vi "Simulador Circuito RLC.Final- Gullit e Gabriela.vi"() -> ()   [LabVIEW 2020]
uses:
  <vilib>/Utility/file.llb/Read Delimited Spreadsheet (DBL).vi
  <vilib>/measure/NI_MABase.lvlib
panel:
  in  "i'(0)":dbl=1.0
  in  "i(0)":dbl
  in  "Vc'(0)":dbl=1.0
  in  "Vc(0)":dbl
  in  "C":dbl
  in  "L":dbl
  in  "R":dbl
  in  "Gerar ondas\nde saída":bool
  out "Tensão no Capacitor":cluster{dbl[], "Y":dbl[]}[](graph)
  out "Corrente":cluster{dbl[], "Y":dbl[]}[](graph)
  in  "Arquivo texto da onda":path
  out "Onda de entrada":cluster{dbl[], "Y":dbl[]}(graph)
  in  "Duty Cicle":dbl
  in  "Informação da amostragem":T1={"Taxa de amostragem"=1000.0, "N° de amostras"=10000.0} {"N° de amostras" format="%#.6g"; "Taxa de amostragem" format="%#.6g"}
  in  "Gerar onda \nde Entrada":bool
  in  "Tipo de Onda":u16(ring) items=["Senoidal", "Quadrada", "Onda qualquer", ""]
  in  "Amplitude":dbl
  in  "Frequência":dbl
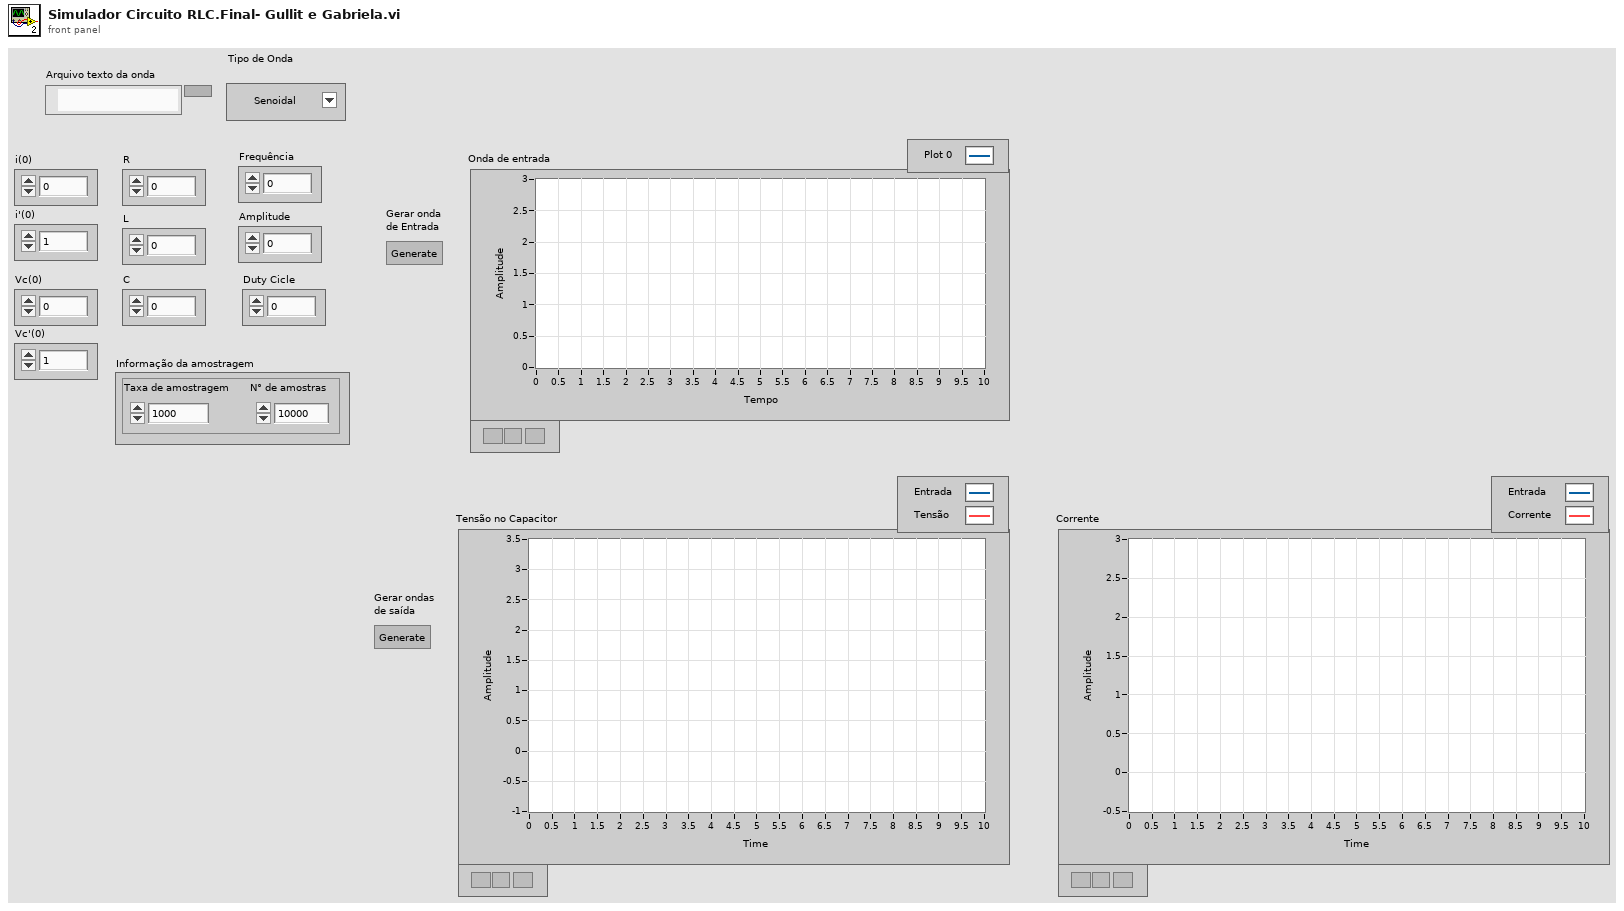
[diagram p1: front panel]
types:
  T1 = cluster{"Taxa de amostragem":dbl, "N° de amostras":dbl}
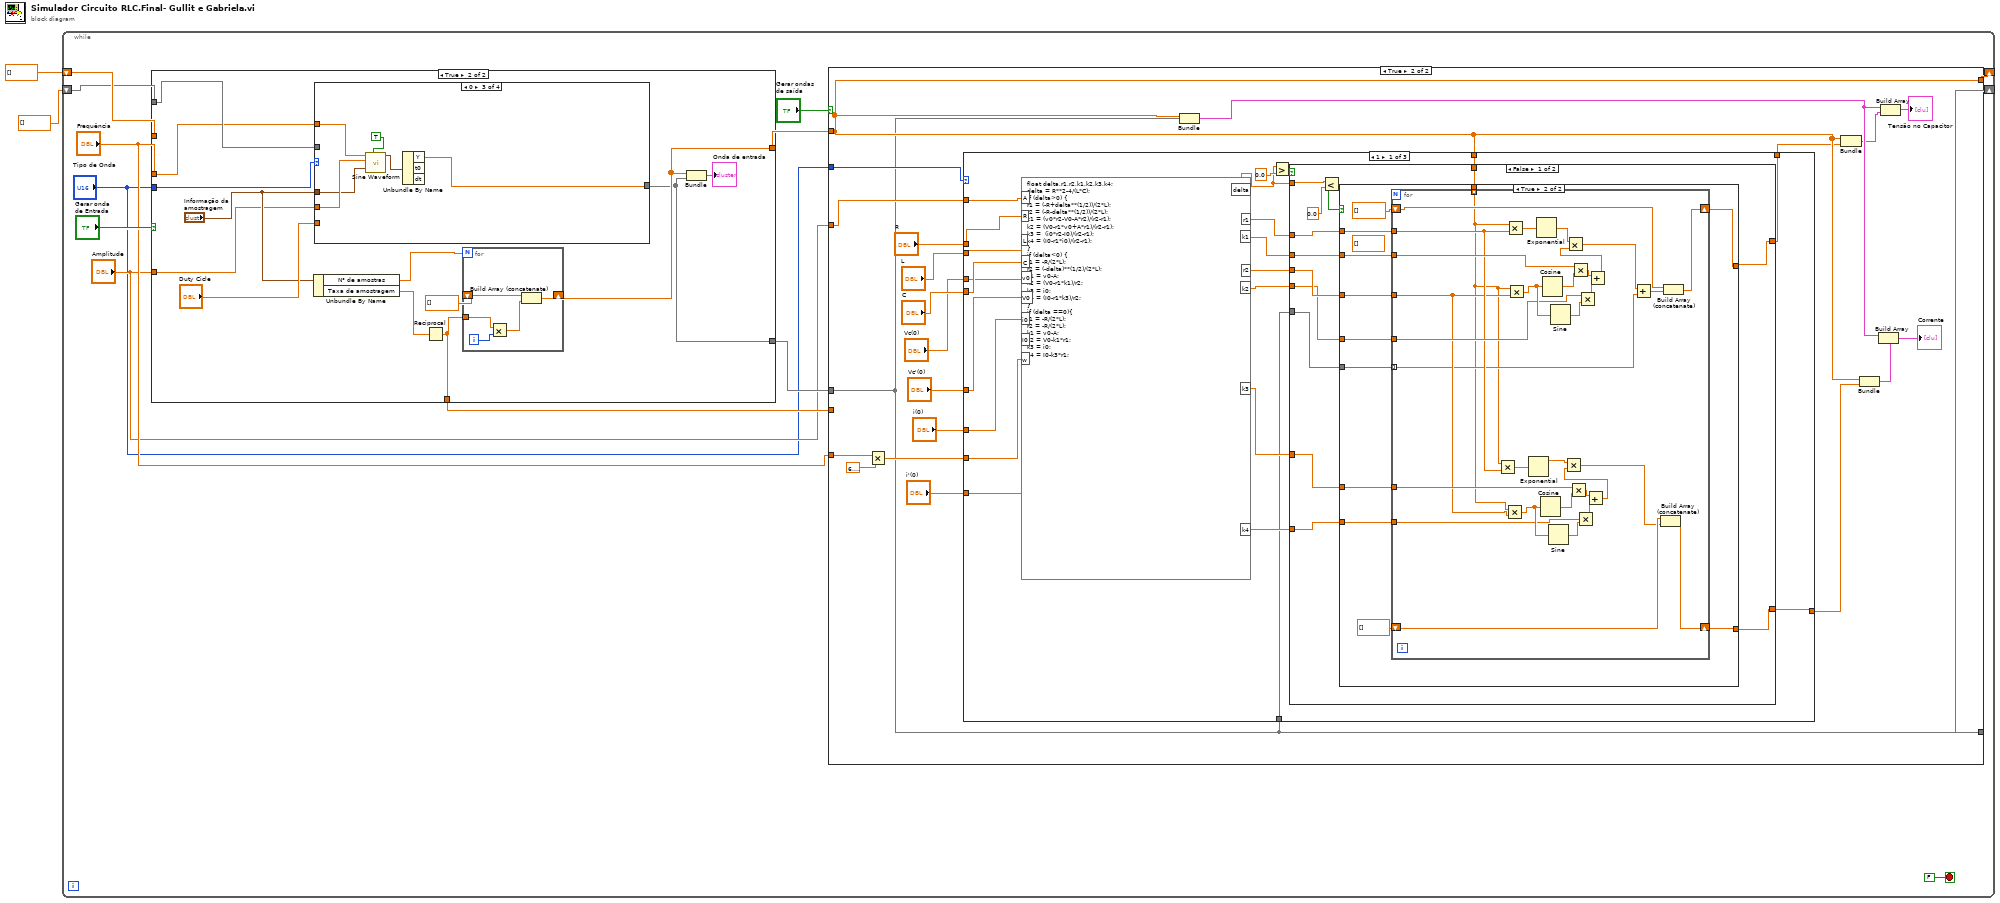
[diagram p0: block diagram]
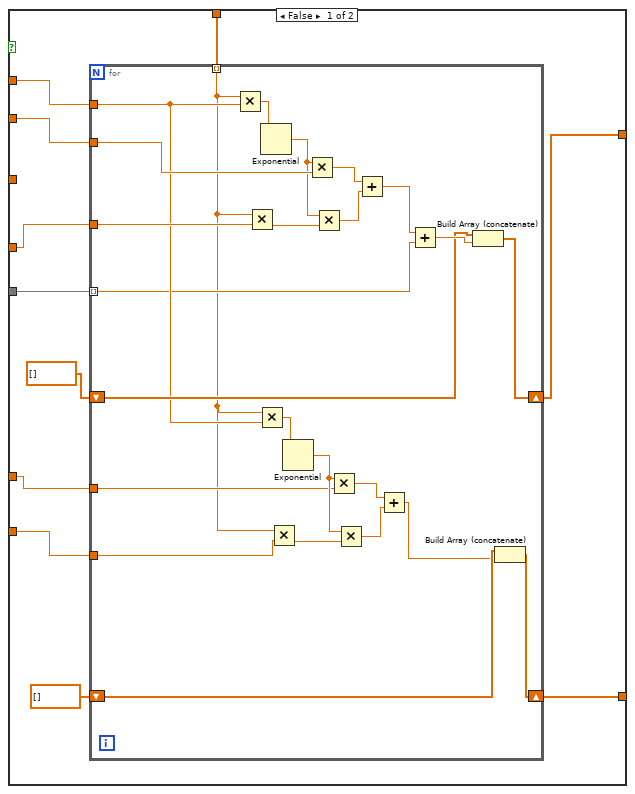
[diagram p3: hidden frame]
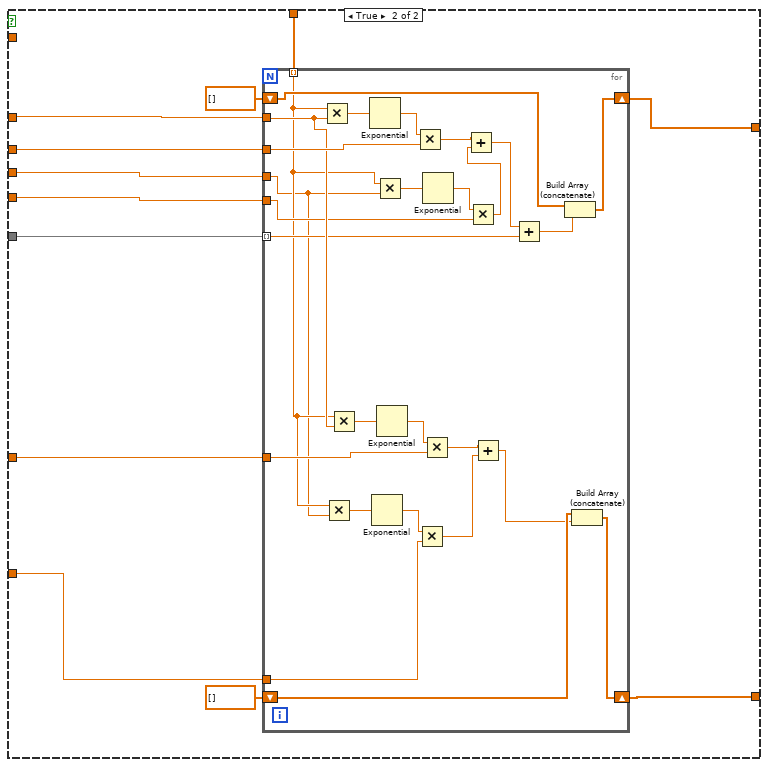
[diagram p4: hidden frame]
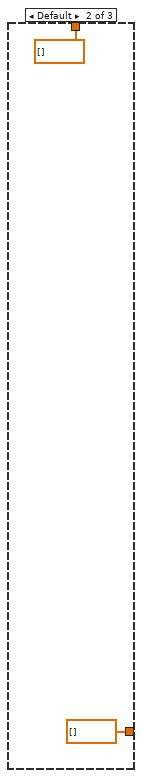
[diagram p5: hidden frame]
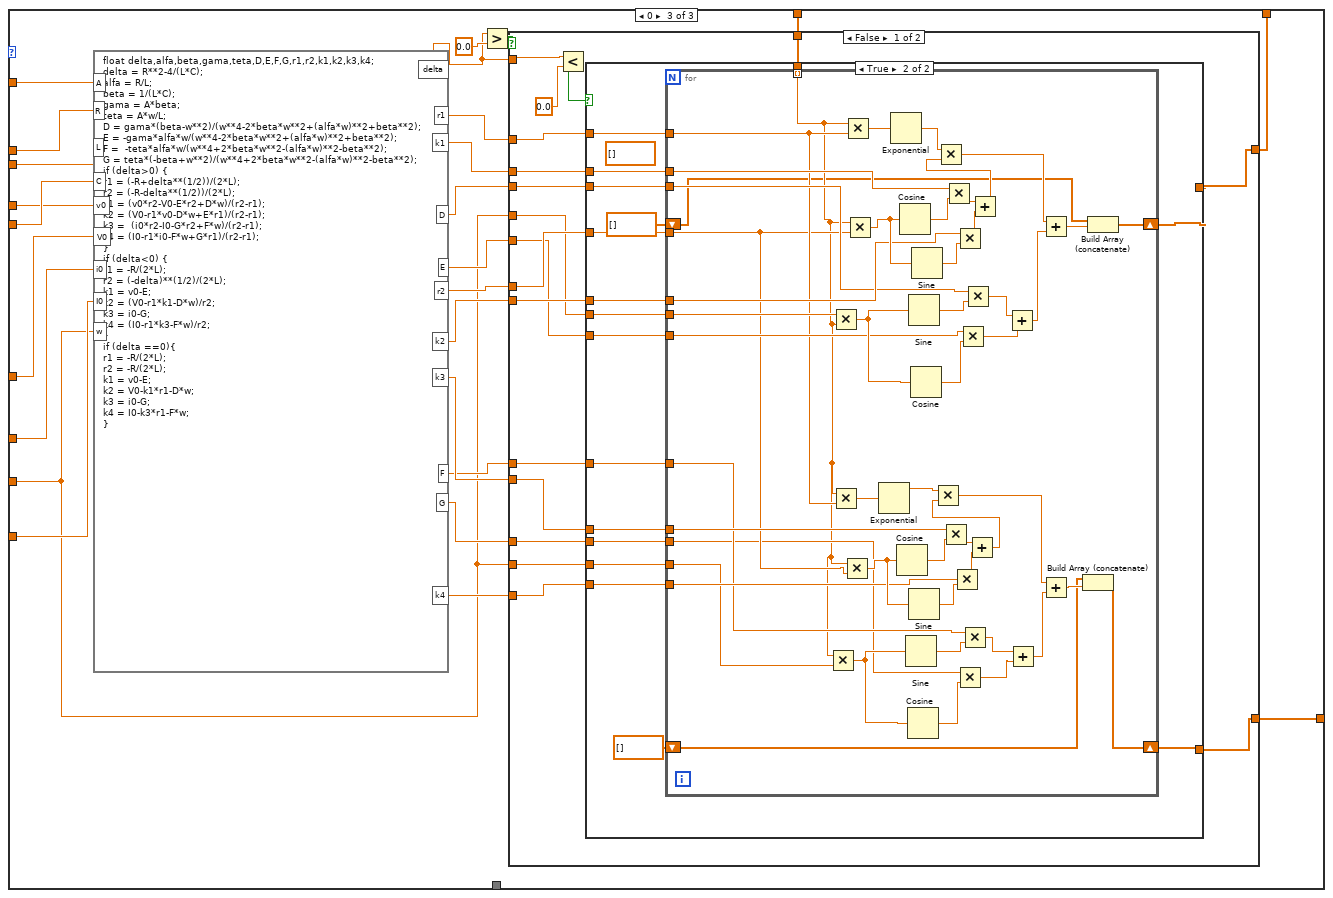
[diagram p6: hidden frame]
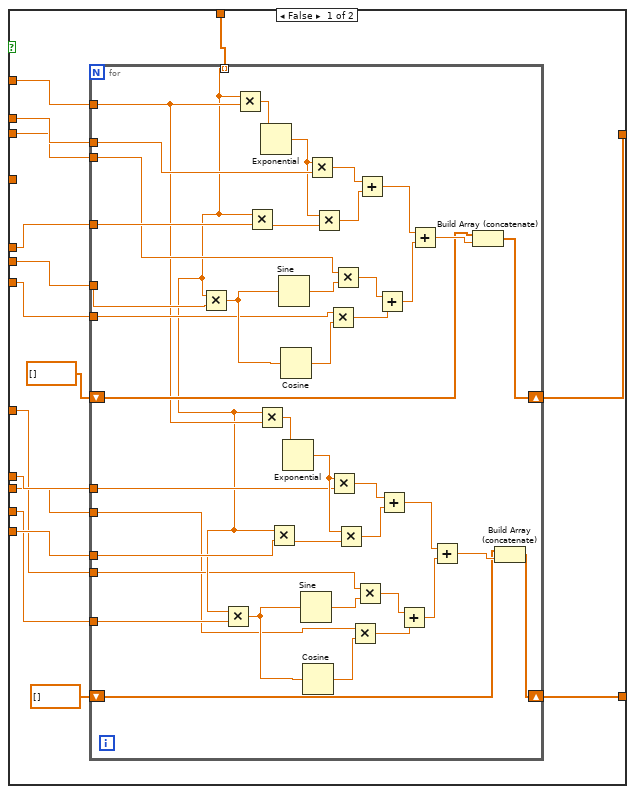
[diagram p7: hidden frame]
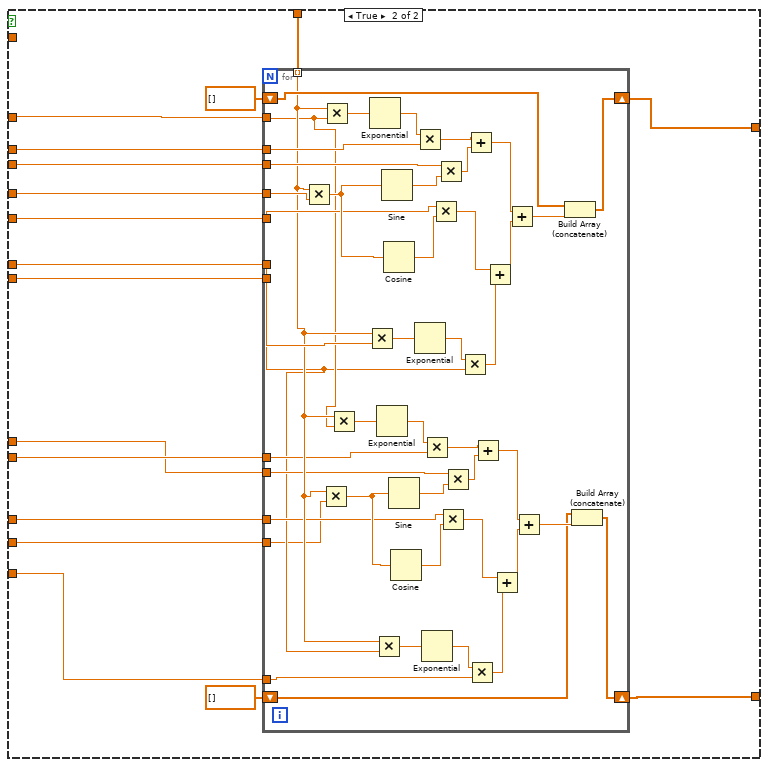
[diagram p8: hidden frame]
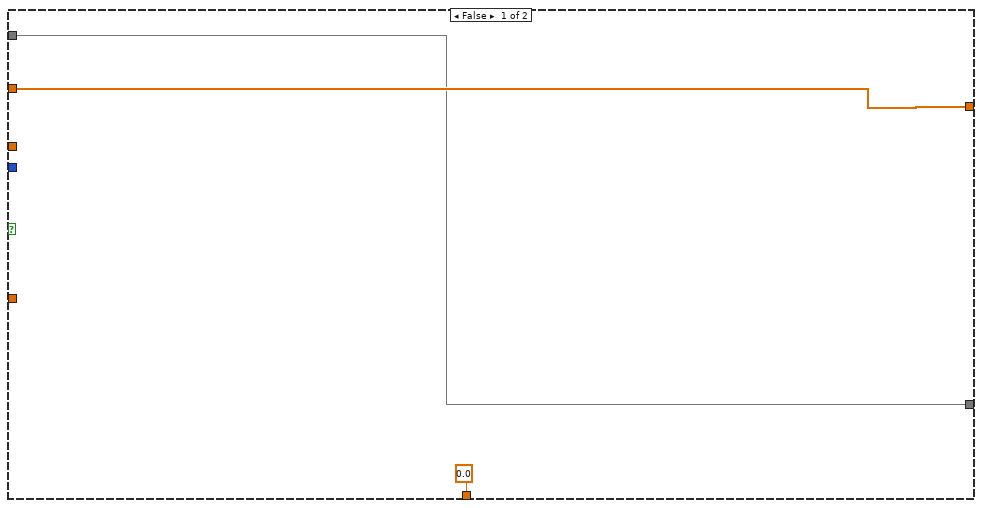
[diagram p9: hidden frame]
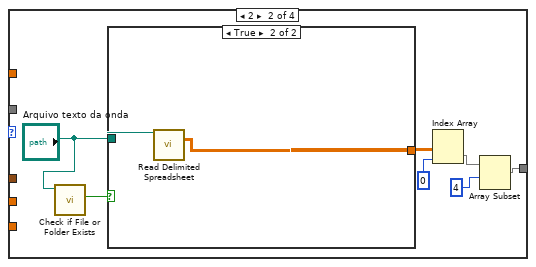
[diagram p11: hidden frame]
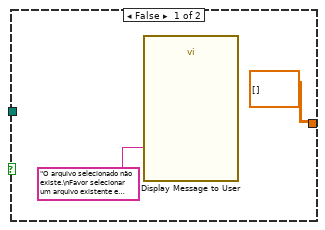
[diagram p12: hidden frame]
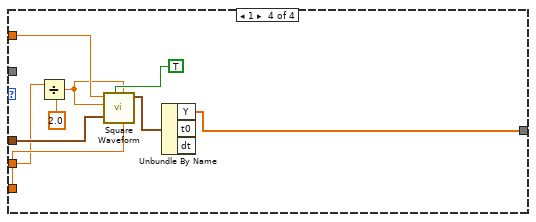
[diagram p13: hidden frame]
diagram:
  n1 = while {
    shift-right: [w11] -> _
    shift-left: dbl[] [] -> [w9]
    shift-right: [w10] -> _
    shift-left: dbl[] [] ("Y") -> [w8]
    stop <- FALSE stop-if-true
    n2 = case shown="True" "Gerar onda \nde Entrada" {
      tunnel: [w424 w432] -> w13
      tunnel: [w423 w431] -> w12
      tunnel: w9 -> [w424 _]
      tunnel: w8 -> [w423 w430]
      tunnel: [0.0 w428] -> w7
      tunnel: "Frequência" -> [_ w427]
      tunnel: "Amplitude" -> [_ w426]
      tunnel: "Tipo de Onda" -> [_ w425]
      frame False {
      }
      frame True {
        n3 = Unbundle By Name("Informação da amostragem") -> ("N° de amostras"=w434:dbl, "Taxa de amostragem"=w435:dbl)
        n4 = case shown="0" w425 {
          tunnel: w426 -> [_ _ w459 w462]
          tunnel: w427 -> [_ _ w460 w469]
          tunnel: w430 -> [w443 _ _ _]
          tunnel: "Informação da amostragem" -> [_ _ w458 w468]
          tunnel: "Duty Cicle" -> [_ _ _ w467]
          tunnel: [w443 w446 w455 w464] -> w431
          frame Default {
          }
          frame 2 {
            n5 = call <vilib>:"Check if File or Folder Exists.vi"("path"="Arquivo texto da onda") -> ("file or folder exists?"=w444:bool)  [unwired: 8 in, 2 out]
            n6 = case shown="True" w444 {
              tunnel: "Arquivo texto da onda" -> [_ w454]
              tunnel: [dbl[][] [] ("all rows") w453] -> w448
              frame False {
                n7 = call "Display Message to User"("Message"="O arquivo selecionado não existe.\nFavor selecionar um arquivo existente e recomeçe a VI.") -> ()  [unwired: 9 in, 2 out]
              }
              frame True {
                n8 = call-poly <vilib>:"Read Delimited Spreadsheet.vi"("file path (dialog if empty)"=w454) -> ("all rows"=w453:dbl[][])  [unwired: 9 in, 5 out]
              }
            }
            n9 = Index Array(array=w448, index (col)=0 ("disabled index (col)")) -> (element=w449:dbl[])  [unwired: 1 in]
            n10 = Array Subset(array=w449, index=4) -> (w446:dbl[])  [unwired: 1 in]
          }
          frame 0 {
            n11 = call <vilib>:"Sine Waveform.vi"("sampling info"=w458, "reset signal"=TRUE, "amplitude"=w459, "frequency"=w460) -> ("signal out"=w456:waveform(dbl))  [unwired: 6 in, 1 out]
            n12 = Unbundle By Name(w456) -> ("Y"=w455:dbl[])  [unwired: 2 out]
          }
          frame 1 {
            n13 = Divide(x=w462, y=2.0) -> (x/y=w461:dbl)
            n14 = call <vilib>:"Square Waveform.vi"("duty cycle (%)"=w467, "offset"=w461, "sampling info"=w468, "reset signal"=TRUE, "amplitude"=w461, "frequency"=w469) -> ("signal out"=w465:waveform(dbl))  [unwired: 4 in, 1 out]
            n15 = Unbundle By Name(w465) -> ("Y"=w464:dbl[])  [unwired: 2 out]
          }
        }
        n16 = Reciprocal(x=w435) -> (1/x=w428:dbl)
        n17 = for {
          N: w434 -> [_]
          tunnel: w428 -> [w441]
          shift-right: [w439] -> w432
          shift-left: dbl[] [] -> [w438]
          i -> [w442]
          n18 = Multiply(x=w441, y=w442) -> (x*y=w440:dbl)
          n19 = Build Array (concatenate)(w438, w440) -> (w439:dbl[])
        }
        n20 = Bundle(w432, "Y"=w431) -> (→"Onda de entrada":cluster{dbl[], "Y":dbl[]})  [unwired: 1 in]
      }
    }
    n21 = case shown="True" "Gerar ondas\nde saída" {
      tunnel: w13 -> [w17 w30]
      tunnel: w12 -> [w16 w18]
      tunnel: [w17 w30] -> w11
      tunnel: [w16 w18] -> w10
      tunnel: w7 -> [_ _]
      tunnel: "Amplitude" -> [_ w20]
      tunnel: "Frequência" -> [_ w22]
      tunnel: "Tipo de Onda" -> [_ w19]
      frame False {
      }
      frame True {
        n22 = Multiply(x=w22, y=6.283185307179586) -> (x*y=w21:dbl)
        n23 = case shown="1" w19 {
          tunnel: "C" -> [w48 _ w217]
          tunnel: "L" -> [w49 _ w216]
          tunnel: "R" -> [w50 _ w215]
          tunnel: "Vc(0)" -> [w47 _ w212]
          tunnel: "Vc'(0)" -> [w46 _ w211]
          tunnel: w30 -> [w42 _ w210]
          tunnel: "i(0)" -> [w45 _ w203]
          tunnel: "i'(0)" -> [w43 _ w202]
          tunnel: [w40 dbl[] [] w196] -> w27
          tunnel: [w41 dbl[] [] w195] -> w26
          tunnel: w21 -> [w44 _ w194]
          tunnel: w20 -> [w51 _ w193]
          tunnel: w18 -> [w39 _ _]
          frame 1 {
            n24 = formula code="float delta,r1,r2,k1,k2,k3,k4;\ndelta = R**2-4/(L*C);\nif (delta>0) {\nr1 = (-R+delta**(1/2))/(2*L);\nr2 = (-R-delta**(1/2))/(2*L);\nk1 = (v0*r2-V0-A*r2)/(r2-r1);\nk2 = (V0-r1*v0+A*r1)/(r2-r1);\nk3 =  (i0*r2-I0)/(r2-r1);\nk4 = (I0-r1*i0)/(r2-r1);\n}\nif (delta<0) {\nr1 = -R/(2*L);\nr2 = (-delta)**(1/2)/(2*L);\nk1 = v0-A;\nk2 = (V0-r1*k1)/r2;\nk3 = i0;\nk4 = (I0-r1*k3)/r2;\n}\nif (delta ==0){\nr1 = -R/(2*L);\nr2 = -R/(2*L);\nk1 = v0-A;\nk2 = V0-k1*r1;\nk3 = i0;\nk4 = I0-k3*r1;\n}"("C"=w48, "L"=w49, "R"=w50, "A"=w51, "w"=w44, "v0"=w47, "V0"=w46, "i0"=w45, "I0"=w43) -> ("delta"=w52:dbl, "r1"=w58:dbl, "r2"=w56:dbl, "k1"=w57:dbl, "k2"=w55:dbl, "k3"=w54:dbl, "k4"=w53:dbl)
            n25 = Greater?(x=w52, y=0.0) -> (0:w59:bool)
            n26 = case shown="False" w59 {
              tunnel: w58 -> [w70 w163]
              tunnel: w57 -> [w69 w162]
              tunnel: w56 -> [w68 w161]
              tunnel: w55 -> [w67 w160]
              tunnel: w54 -> [w66 w158]
              tunnel: w53 -> [w65 w157]
              tunnel: w52 -> [w72 _]
              tunnel: [w63 w155] -> w40
              tunnel: [w64 w154] -> w41
              tunnel: w42 -> [w62 w153]
              tunnel: w39 -> [w61 w152]
              frame False {
                n27 = Less?(x=w72, y=0.0) -> (x < y?=w73:bool)
                n28 = case shown="True" w73 {
                  tunnel: w70 -> [w83 w120]
                  tunnel: w69 -> [w84 w119]
                  tunnel: w68 -> [_ w118]
                  tunnel: w67 -> [w82 w117]
                  tunnel: w66 -> [w80 w116]
                  tunnel: w65 -> [w79 w115]
                  tunnel: [w74 w109] -> w63
                  tunnel: [w77 w113] -> w64
                  tunnel: w62 -> [w76 w111]
                  tunnel: w61 -> [w75 w110]
                  frame False {
                    n29 = for {
                      tunnel: w84 -> [w108]
                      tunnel: w83 -> [w92]
                      tunnel: w82 -> [w106]
                      shift-right: [w99] -> w74
                      shift-left: dbl[] [] -> [w98]
                      tunnel: w80 -> [w91]
                      tunnel: w79 -> [w90]
                      shift-right: [w89] -> w77
                      shift-left: dbl[] [] -> [w88]
                      tunnel: w76 -> [w86] mode=indexing
                      tunnel: w75 -> [w87] mode=indexing
                      n30 = Multiply(x=w86, y=w92) -> (x*y=w107:dbl)
                      n31 = Multiply(x=w86, y=w106) -> (x*y=w105:dbl)
                      n32 = Multiply(x=w86, y=w92) -> (x*y=w97:dbl)
                      n33 = Exponential(1:w107) -> (0:w104:dbl)
                      n34 = Multiply(x=w86, y=w90) -> (x*y=w96:dbl)
                      n35 = Exponential(1:w97) -> (0:w95:dbl)
                      n36 = Multiply(x=w104, y=w108) -> (x*y=w103:dbl)
                      n37 = Multiply(x=w104, y=w105) -> (x*y=w102:dbl)
                      n38 = Multiply(x=w95, y=w91) -> (x*y=w94:dbl)
                      n39 = Multiply(x=w95, y=w96) -> (x*y=w93:dbl)
                      n40 = Add(x=w103, y=w102) -> (x+y=w101:dbl)
                      n41 = Add(x=w94, y=w93) -> (x+y=w85:dbl)
                      n42 = Add(x=w101, y=w87) -> (x+y=w100:dbl)
                      n43 = Build Array (concatenate)(w98, w100) -> (w99:dbl[])
                      n44 = Build Array (concatenate)(w88, w85) -> (w89:dbl[])
                    }
                  }
                  frame True {
                    (unwired) dbl[] []
                    n45 = for {
                      tunnel: w120 -> [w139]
                      tunnel: w119 -> [w147]
                      tunnel: w118 -> [w129]
                      tunnel: w117 -> [w143]
                      tunnel: w116 -> [w132]
                      tunnel: w115 -> [w131]
                      shift-right: [w127] -> w113
                      shift-left: dbl[] [] -> [w126]
                      shift-right: [w125] -> w109
                      shift-left: dbl[] [] -> [w124]
                      tunnel: w111 -> [w122] mode=indexing
                      tunnel: w110 -> [w123] mode=indexing
                      n46 = Multiply(x=w122, y=w139) -> (x*y=w148:dbl)
                      n47 = Multiply(x=w122, y=w129) -> (x*y=w137:dbl)
                      n48 = Multiply(x=w122, y=w139) -> (x*y=w151:dbl)
                      n49 = Multiply(x=w122, y=w129) -> (x*y=w145:dbl)
                      n50 = Exponential(1:w148) -> (0:w133:dbl)
                      n51 = Exponential(1:w151) -> (0:w150:dbl)
                      n52 = Cosine(x=w137) -> (cos(x)=w138:dbl)
                      n53 = Cosine(x=w145) -> (cos(x)=w146:dbl)
                      n54 = Sine(x=w137) -> (sin(x)=w136:dbl)
                      n55 = Sine(x=w145) -> (sin(x)=w144:dbl)
                      n56 = Multiply(x=w132, y=w138) -> (x*y=w135:dbl)
                      n57 = Multiply(x=w147, y=w146) -> (x*y=w142:dbl)
                      n58 = Multiply(x=w131, y=w136) -> (x*y=w134:dbl)
                      n59 = Multiply(x=w143, y=w144) -> (x*y=w141:dbl)
                      n60 = Add(x=w135, y=w134) -> (x+y=w130:dbl)
                      n61 = Multiply(x=w133, y=w130) -> (x*y=w121:dbl)
                      n62 = Add(x=w142, y=w141) -> (x+y=w140:dbl)
                      n63 = Multiply(x=w150, y=w140) -> (x*y=w128:dbl)
                      n64 = Add(x=w128, y=w123) -> (x+y=w149:dbl)
                      n65 = Build Array (concatenate)(w126, w121) -> (w127:dbl[])
                      n66 = Build Array (concatenate)(w124, w149) -> (w125:dbl[])
                    }
                  }
                }
              }
              frame True {
                n67 = for {
                  tunnel: w163 -> [w175]
                  tunnel: w162 -> [w190]
                  tunnel: w161 -> [w167]
                  tunnel: w160 -> [w171]
                  shift-right: [w182] -> w155
                  shift-left: dbl[] [] -> [w181]
                  tunnel: w158 -> [w174]
                  tunnel: w157 -> [w166]
                  shift-right: [w173] -> w154
                  shift-left: dbl[] [] -> [w172]
                  tunnel: w153 -> [w168] mode=indexing
                  tunnel: w152 -> [w169] mode=indexing
                  n68 = Multiply(x=w168, y=w175) -> (x*y=w189:dbl)
                  n69 = Multiply(x=w168, y=w167) -> (x*y=w178:dbl)
                  n70 = Multiply(x=w168, y=w175) -> (x*y=w180:dbl)
                  n71 = Exponential(1:w189) -> (0:w188:dbl)
                  n72 = Exponential(1:w178) -> (0:w177:dbl)
                  n73 = Multiply(x=w168, y=w167) -> (x*y=w187:dbl)
                  n74 = Exponential(1:w180) -> (0:w179:dbl)
                  n75 = Multiply(x=w188, y=w190) -> (x*y=w185:dbl)
                  n76 = Multiply(x=w177, y=w166) -> (x*y=w165:dbl)
                  n77 = Multiply(x=w179, y=w174) -> (x*y=w176:dbl)
                  n78 = Exponential(1:w187) -> (0:w186:dbl)
                  n79 = Multiply(x=w186, y=w171) -> (x*y=w170:dbl)
                  n80 = Add(x=w185, y=w170) -> (x+y=w184:dbl)
                  n81 = Add(x=w176, y=w165) -> (x+y=w164:dbl)
                  n82 = Add(x=w184, y=w169) -> (x+y=w183:dbl)
                  n83 = Build Array (concatenate)(w181, w183) -> (w182:dbl[])
                  n84 = Build Array (concatenate)(w172, w164) -> (w173:dbl[])
                }
              }
            }
          }
          frame Default {
          }
          frame 0 {
            n85 = formula code="float delta,alfa,beta,gama,teta,D,E,F,G,r1,r2,k1,k2,k3,k4;\ndelta = R**2-4/(L*C);\nalfa = R/L;\nbeta = 1/(L*C);\ngama = A*beta;\nteta = A*w/L;\nD = gama*(beta-w**2)/(w**4-2*beta*w**2+(alfa*w)**2+beta**2);\nE = -gama*alfa*w/(w**4-2*beta*w**2+(alfa*w)**2+beta**2);\nF =  -teta*alfa*w/(w**4+2*beta*w**2-(alfa*w)**2-beta**2);\nG = teta*(-beta+w**2)/(w**4+2*beta*w**2-(alfa*w)**2-beta**2);\nif (delta>0) {\nr1 = (-R+delta**(1/2))/(2*L);\nr2 = (-R-delta**(1/2))/(2*L);\nk1 = (v0*r2-V0-E*r2+D*w)/(r2-r1);\nk2 = (V0-r1*v0-D*w+E*r1)/(r2-r1);\nk3 =  (i0*r2-I0-G*r2+F*w)/(r2-r1);\nk4 = (I0-r1*i0-F*w+G*r1)/(r2-r1);\n}\nif (delta<0) {\nr1 = -R/(2*L);\nr2 = (-delta)**(1/2)/(2*L);\nk1 = v0-E;\nk2 = (V0-r1*k1-D*w)/r2;\nk3 = i0-G;\nk4 = (I0-r1*k3-F*w)/r2;\n}\nif (delta ==0){\nr1 = -R/(2*L);\nr2 = -R/(2*L);\nk1 = v0-E;\nk2 = V0-k1*r1-D*w;\nk3 = i0-G;\nk4 = I0-k3*r1-F*w;\n}"("C"=w217, "L"=w216, "R"=w215, "A"=w193, "w"=w194, "v0"=w212, "V0"=w211, "i0"=w203, "I0"=w202) -> ("D"=w204:dbl, "E"=w205:dbl, "delta"=w197:dbl, "r1"=w209:dbl, "r2"=w207:dbl, "k1"=w208:dbl, "k2"=w206:dbl, "k3"=w201:dbl, "k4"=w198:dbl, "F"=w200:dbl, "G"=w199:dbl)
            n86 = Greater?(x=w197, y=0.0) -> (0:w213:bool)
            n87 = case shown="False" w213 {
              tunnel: w210 -> [w232 w376]
              tunnel: w209 -> [w231 w375]
              tunnel: w208 -> [w230 w374]
              tunnel: w207 -> [w229 w373]
              tunnel: w206 -> [w228 w372]
              tunnel: w194 -> [w227 w371]
              tunnel: w205 -> [w225 w370]
              tunnel: w204 -> [w226 w369]
              tunnel: w201 -> [w224 w367]
              tunnel: w200 -> [w221 w366]
              tunnel: w199 -> [w220 w365]
              tunnel: w198 -> [w222 w364]
              tunnel: w194 -> [w223 w362]
              tunnel: w197 -> [w234 _]
              tunnel: [w218 w361] -> w196
              tunnel: [w219 w360] -> w195
              frame False {
                n88 = Less?(x=w234, y=0.0) -> (x < y?=w235:bool)
                n89 = case shown="True" w235 {
                  tunnel: w232 -> [w250 w307]
                  tunnel: w231 -> [w249 w310]
                  tunnel: w230 -> [w251 w309]
                  tunnel: w229 -> [_ w308]
                  tunnel: w228 -> [w248 w306]
                  tunnel: w227 -> [w247 w305]
                  tunnel: w226 -> [w246 w304]
                  tunnel: w225 -> [w245 w303]
                  tunnel: w224 -> [w243 w302]
                  tunnel: w223 -> [w241 w301]
                  tunnel: w222 -> [w242 w300]
                  tunnel: w221 -> [w240 w299]
                  tunnel: w220 -> [w239 w298]
                  tunnel: [w237 w294] -> w218
                  tunnel: [w236 w296] -> w219
                  frame False {
                    n90 = for {
                      tunnel: w251 -> [w293]
                      tunnel: w250 -> [w256] mode=indexing
                      tunnel: w249 -> [w260]
                      tunnel: w248 -> [w291]
                      tunnel: w247 -> [w281]
                      tunnel: w246 -> [w280]
                      tunnel: w245 -> [w279]
                      shift-right: [w275] -> w237
                      shift-left: dbl[] [] -> [w274]
                      tunnel: w243 -> [w259]
                      tunnel: w242 -> [w258]
                      tunnel: w241 -> [w257]
                      tunnel: w240 -> [w255]
                      tunnel: w239 -> [w254]
                      shift-right: [w253] -> w236
                      shift-left: dbl[] [] -> [w252]
                      n91 = Multiply(x=w256, y=w281) -> (x*y=w286:dbl)
                      n92 = Multiply(x=w256, y=w257) -> (x*y=w268:dbl)
                      n93 = Multiply(x=w256, y=w260) -> (x*y=w292:dbl)
                      n94 = Multiply(x=w256, y=w291) -> (x*y=w290:dbl)
                      n95 = Multiply(x=w256, y=w260) -> (x*y=w273:dbl)
                      n96 = Exponential(1:w292) -> (0:w289:dbl)
                      n97 = Multiply(x=w256, y=w258) -> (x*y=w272:dbl)
                      n98 = Sine(x=w286) -> (sin(x)=w284:dbl)
                      n99 = Cosine(x=w286) -> (cos(x)=w285:dbl)
                      n100 = Exponential(1:w273) -> (0:w271:dbl)
                      n101 = Sine(x=w268) -> (sin(x)=w266:dbl)
                      n102 = Cosine(x=w268) -> (cos(x)=w267:dbl)
                      n103 = Multiply(x=w289, y=w293) -> (x*y=w288:dbl)
                      n104 = Multiply(x=w289, y=w290) -> (x*y=w287:dbl)
                      n105 = Multiply(x=w279, y=w285) -> (x*y=w283:dbl)
                      n106 = Multiply(x=w271, y=w259) -> (x*y=w270:dbl)
                      n107 = Multiply(x=w280, y=w284) -> (x*y=w282:dbl)
                      n108 = Multiply(x=w271, y=w272) -> (x*y=w269:dbl)
                      n109 = Multiply(x=w254, y=w267) -> (x*y=w265:dbl)
                      n110 = Multiply(x=w255, y=w266) -> (x*y=w264:dbl)
                      n111 = Add(x=w288, y=w287) -> (x+y=w278:dbl)
                      n112 = Add(x=w282, y=w283) -> (x+y=w277:dbl)
                      n113 = Add(x=w270, y=w269) -> (x+y=w263:dbl)
                      n114 = Add(x=w264, y=w265) -> (x+y=w262:dbl)
                      n115 = Add(x=w278, y=w277) -> (x+y=w276:dbl)
                      n116 = Add(x=w263, y=w262) -> (x+y=w261:dbl)
                      n117 = Build Array (concatenate)(w274, w276) -> (w275:dbl[])
                      n118 = Build Array (concatenate)(w252, w261) -> (w253:dbl[])
                    }
                  }
                  frame True {
                    (unwired) dbl[] []
                    n119 = for {
                      tunnel: w310 -> [w340]
                      tunnel: w309 -> [w351]
                      tunnel: w308 -> [w327]
                      tunnel: w307 -> [w313] mode=indexing
                      tunnel: w306 -> [w347]
                      tunnel: w305 -> [w343]
                      tunnel: w304 -> [w342]
                      tunnel: w303 -> [w341]
                      tunnel: w302 -> [w330]
                      tunnel: w301 -> [w326]
                      tunnel: w300 -> [w329]
                      tunnel: w299 -> [w325]
                      tunnel: w298 -> [w324]
                      shift-right: [w315] -> w296
                      shift-left: dbl[] [] -> [w314]
                      shift-right: [w312] -> w294
                      shift-left: dbl[] [] -> [w311]
                      n120 = Multiply(x=w313, y=w326) -> (x*y=w339:dbl)
                      n121 = Multiply(x=w343, y=w313) -> (x*y=w357:dbl)
                      n122 = Multiply(x=w313, y=w340) -> (x*y=w352:dbl)
                      n123 = Multiply(x=w313, y=w327) -> (x*y=w335:dbl)
                      n124 = Multiply(x=w313, y=w340) -> (x*y=w359:dbl)
                      n125 = Multiply(x=w313, y=w327) -> (x*y=w349:dbl)
                      n126 = Exponential(1:w352) -> (0:w331:dbl)
                      n127 = Exponential(1:w359) -> (0:w358:dbl)
                      n128 = Cosine(x=w335) -> (cos(x)=w336:dbl)
                      n129 = Cosine(x=w349) -> (cos(x)=w350:dbl)
                      n130 = Sine(x=w339) -> (sin(x)=w337:dbl)
                      n131 = Cosine(x=w339) -> (cos(x)=w338:dbl)
                      n132 = Sine(x=w357) -> (sin(x)=w355:dbl)
                      n133 = Sine(x=w335) -> (sin(x)=w334:dbl)
                      n134 = Cosine(x=w357) -> (cos(x)=w356:dbl)
                      n135 = Sine(x=w349) -> (sin(x)=w348:dbl)
                      n136 = Multiply(x=w330, y=w336) -> (x*y=w333:dbl)
                      n137 = Multiply(x=w351, y=w350) -> (x*y=w346:dbl)
                      n138 = Multiply(x=w329, y=w334) -> (x*y=w332:dbl)
                      n139 = Multiply(x=w347, y=w348) -> (x*y=w345:dbl)
                      n140 = Multiply(x=w324, y=w338) -> (x*y=w322:dbl)
                      n141 = Multiply(x=w341, y=w356) -> (x*y=w318:dbl)
                      n142 = Multiply(x=w325, y=w337) -> (x*y=w323:dbl)
                      n143 = Multiply(x=w342, y=w355) -> (x*y=w317:dbl)
                      n144 = Add(x=w333, y=w332) -> (x+y=w328:dbl)
                      n145 = Multiply(x=w331, y=w328) -> (x*y=w320:dbl)
                      n146 = Add(x=w346, y=w345) -> (x+y=w344:dbl)
                      n147 = Multiply(x=w358, y=w344) -> (x*y=w316:dbl)
                      n148 = Add(x=w317, y=w318) -> (x+y=w354:dbl)
                      n149 = Add(x=w323, y=w322) -> (x+y=w321:dbl)
                      n150 = Add(x=w316, y=w354) -> (x+y=w353:dbl)
                      n151 = Add(x=w320, y=w321) -> (x+y=w319:dbl)
                      n152 = Build Array (concatenate)(w314, w319) -> (w315:dbl[])
                      n153 = Build Array (concatenate)(w311, w353) -> (w312:dbl[])
                    }
                  }
                }
              }
              frame True {
                n154 = for {
                  tunnel: w376 -> [w386] mode=indexing
                  tunnel: w375 -> [w385]
                  tunnel: w374 -> [w421]
                  tunnel: w373 -> [w416]
                  tunnel: w372 -> [w380]
                  tunnel: w371 -> [w415]
                  tunnel: w370 -> [w412]
                  tunnel: w369 -> [w410]
                  shift-right: [w402] -> w361
                  shift-left: dbl[] [] -> [w401]
                  tunnel: w367 -> [w384]
                  tunnel: w366 -> [w383]
                  tunnel: w365 -> [w382]
                  tunnel: w364 -> [w381]
                  shift-right: [w379] -> w360
                  shift-left: dbl[] [] -> [w378]
                  tunnel: w362 -> [w377]
                  n155 = Multiply(x=w386, y=w415) -> (x*y=w414:dbl)
                  n156 = Multiply(x=w386, y=w377) -> (x*y=w396:dbl)
                  n157 = Multiply(x=w386, y=w385) -> (x*y=w420:dbl)
                  n158 = Multiply(x=w386, y=w385) -> (x*y=w400:dbl)
                  n159 = Multiply(x=w386, y=w416) -> (x*y=w418:dbl)
                  n160 = Exponential(1:w420) -> (0:w419:dbl)
                  n161 = Multiply(x=w386, y=w380) -> (x*y=w398:dbl)
                  n162 = Exponential(1:w400) -> (0:w399:dbl)
                  n163 = Sine(x=w414) -> (sin(x)=w411:dbl)
                  n164 = Cosine(x=w414) -> (cos(x)=w413:dbl)
                  n165 = Sine(x=w396) -> (sin(x)=w394:dbl)
                  n166 = Cosine(x=w396) -> (cos(x)=w395:dbl)
                  n167 = Multiply(x=w419, y=w421) -> (x*y=w408:dbl)
                  n168 = Exponential(1:w418) -> (0:w417:dbl)
                  n169 = Multiply(x=w399, y=w384) -> (x*y=w392:dbl)
                  n170 = Exponential(1:w398) -> (0:w397:dbl)
                  n171 = Multiply(x=w412, y=w413) -> (x*y=w406:dbl)
                  n172 = Multiply(x=w410, y=w411) -> (x*y=w409:dbl)
                  n173 = Multiply(x=w382, y=w395) -> (x*y=w390:dbl)
                  n174 = Multiply(x=w383, y=w394) -> (x*y=w393:dbl)
                  n175 = Multiply(x=w417, y=w380) -> (x*y=w407:dbl)
                  n176 = Add(x=w408, y=w409) -> (x+y=w404:dbl)
                  n177 = Multiply(x=w397, y=w381) -> (x*y=w391:dbl)
                  n178 = Add(x=w392, y=w393) -> (x+y=w388:dbl)
                  n179 = Add(x=w406, y=w407) -> (x+y=w405:dbl)
                  n180 = Add(x=w390, y=w391) -> (x+y=w389:dbl)
                  n181 = Add(x=w404, y=w405) -> (x+y=w403:dbl)
                  n182 = Add(x=w388, y=w389) -> (x+y=w387:dbl)
                  n183 = Build Array (concatenate)(w401, w403) -> (w402:dbl[])
                  n184 = Build Array (concatenate)(w378, w387) -> (w379:dbl[])
                }
              }
            }
          }
        }
        n185 = Bundle(w30, "Y"=w18) -> (w38:cluster{dbl[], "Y":dbl[]})  [unwired: 1 in]
        n186 = Bundle(w30, w27) -> (w24:cluster{dbl[], dbl[]})  [unwired: 1 in]
        n187 = Bundle(w30, w26) -> (w25:cluster{dbl[], dbl[]})  [unwired: 1 in]
        n188 = Build Array(w38, w25) -> (→"Corrente":cluster{dbl[], "Y":dbl[]}[])
        n189 = Build Array(w38, w24) -> (→"Tensão no Capacitor":cluster{dbl[], "Y":dbl[]}[])
      }
    }
  }
